vi "Periodic Tasks.vi"(8 "error in":errorcluster) -> ()   [LabVIEW 2016]
doc: "This VI runs in parallel to other tasks. It can contain as many user-defined periodic loops as you need. These can carry out PID or other sorts of timed response."
uses:
  <vilib>/Rock Robotics/WPI/Utilities/WPI_GetSetVariantRefNum.vi
  <vilib>/Instr/_visa.llb/VISA Configure Serial Port (Instr).vi
  2_11_17/Systems/Global 1.vi
panel:
  out "Drive L0 Effort":dbl format="%#_13g"
  out "Drive R0 Effort":dbl format="%#_13g"
  in  "off set":dbl=55.0 format="%#_13g"
  out "read buffer":string="B:3,X:197.00,Y:124.00"
  in  "Search_Params":string[](array[string])=["B", "X", "Y", "W1", "H1", "W2", "H2"]
  out "Last Complete Message":string="B:2,X:197.00,Y:124.00,W1:9,H1:24,W2:9,H2:23"
  out "length":i32=43
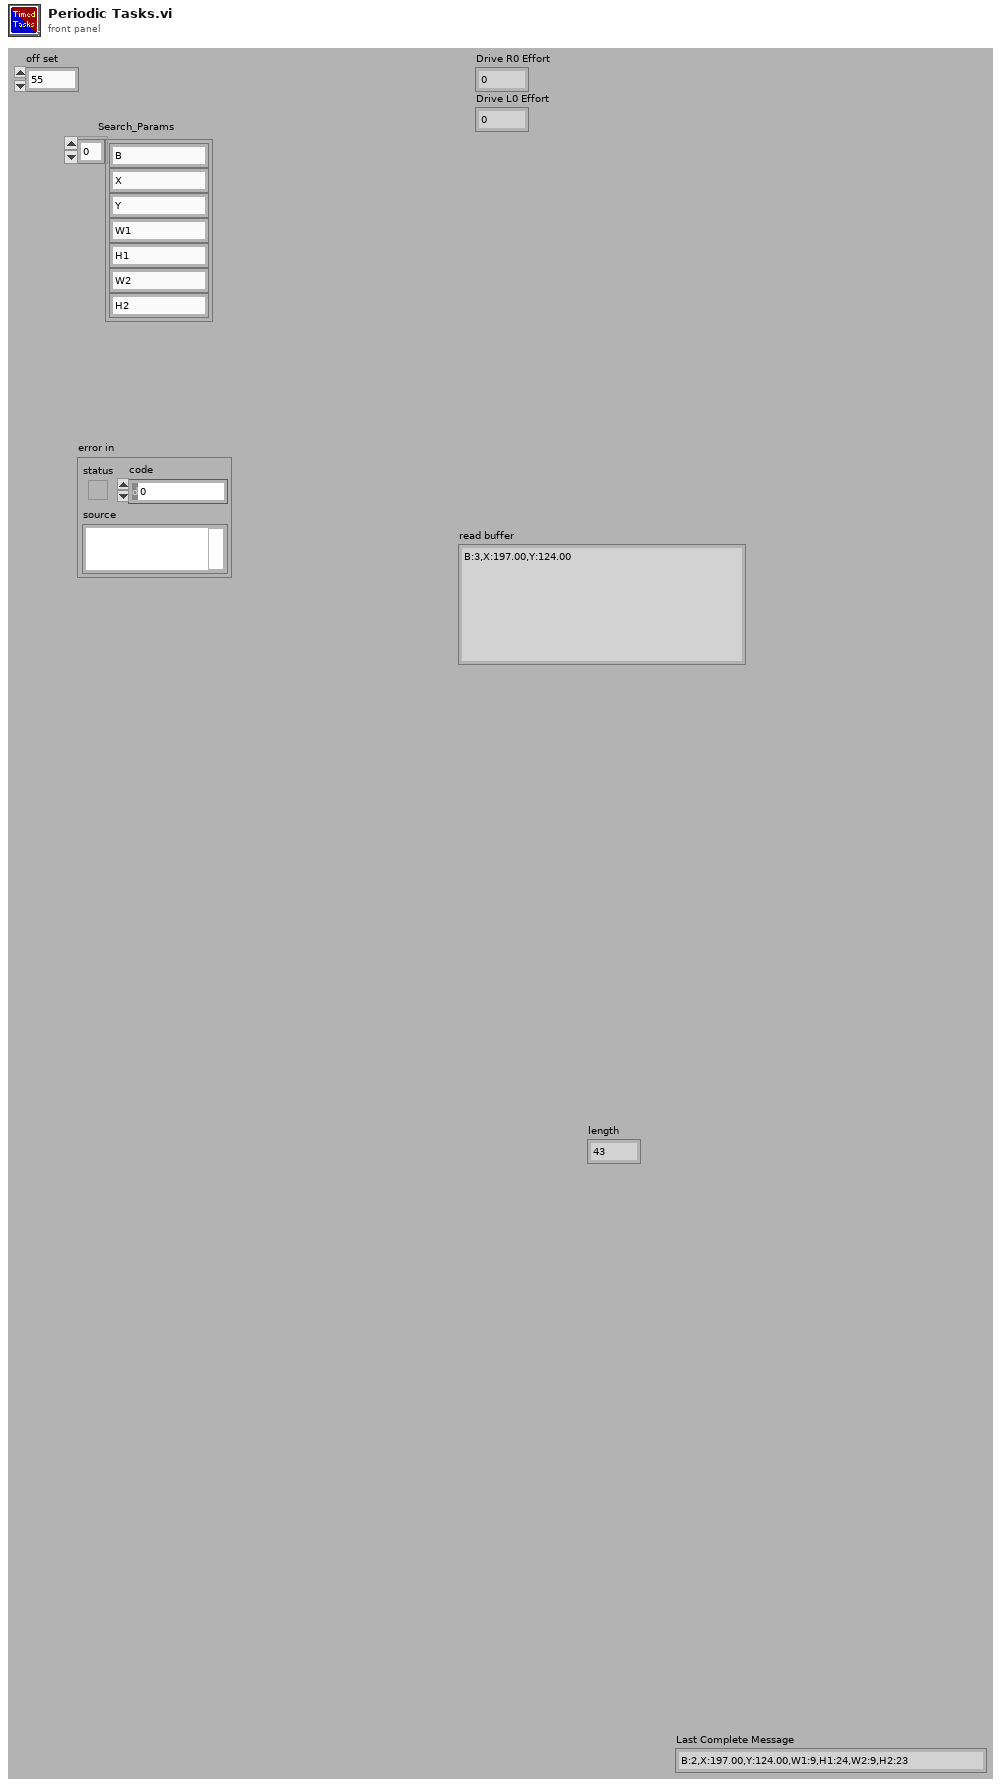
[diagram p1: front panel]
types:
  T1 = typedef "WPI_JoystickDevRef.ctl" = cluster{"Device":T2}
  T2 = typedef "WPI_JoystickDeviceEnum.ctl" = enum16{"USB 0", "USB 1", "USB 2", "USB 3", "USB 4", "USB 5"}
  T3 = typedef "WPI_MotorControlDeviceRef.ctl" = cluster{"DeviceStatus":errorcluster, "Type":T4, "PWM":cluster{"PWM Channel":T5, "DeadBand":T6}, "CAN":cluster{"Device Number":u8, "SetOutput VI Ref":variant, "GetOutput VI Ref":variant, "Enable VI Ref":variant, "Disable VI Ref":variant, "Data":variant}, "Invert":bool}
  T4 = typedef "WPI_MotorControlType.ctl" = enum16{"PWM", "CAN"}
  T5 = typedef "FPGA_DIOPWMChannel.ctl" = enum8{"PWM 0", "PWM 1", "PWM 2", "PWM 3", "PWM 4", "PWM 5", "PWM 6", "PWM 7", "PWM 8", "PWM 9", "PWM MXP 0", "PWM MXP 1", "PWM MXP 2", "PWM MXP 3", "PWM MXP 4", "PWM MXP 5", "PWM MXP 6", "PWM MXP 7", "PWM MXP 8", "PWM MXP 9", "Invalid"}
  T6 = typedef "WPI_PWMDeadband.ctl" = cluster{"Name":string, "maxPositivePwm":i32, "minPositivePwm":i32, "centerPwm":i32, "maxNegativePwm":i32, "minNegativePwm":i32, "angularRange":u16}
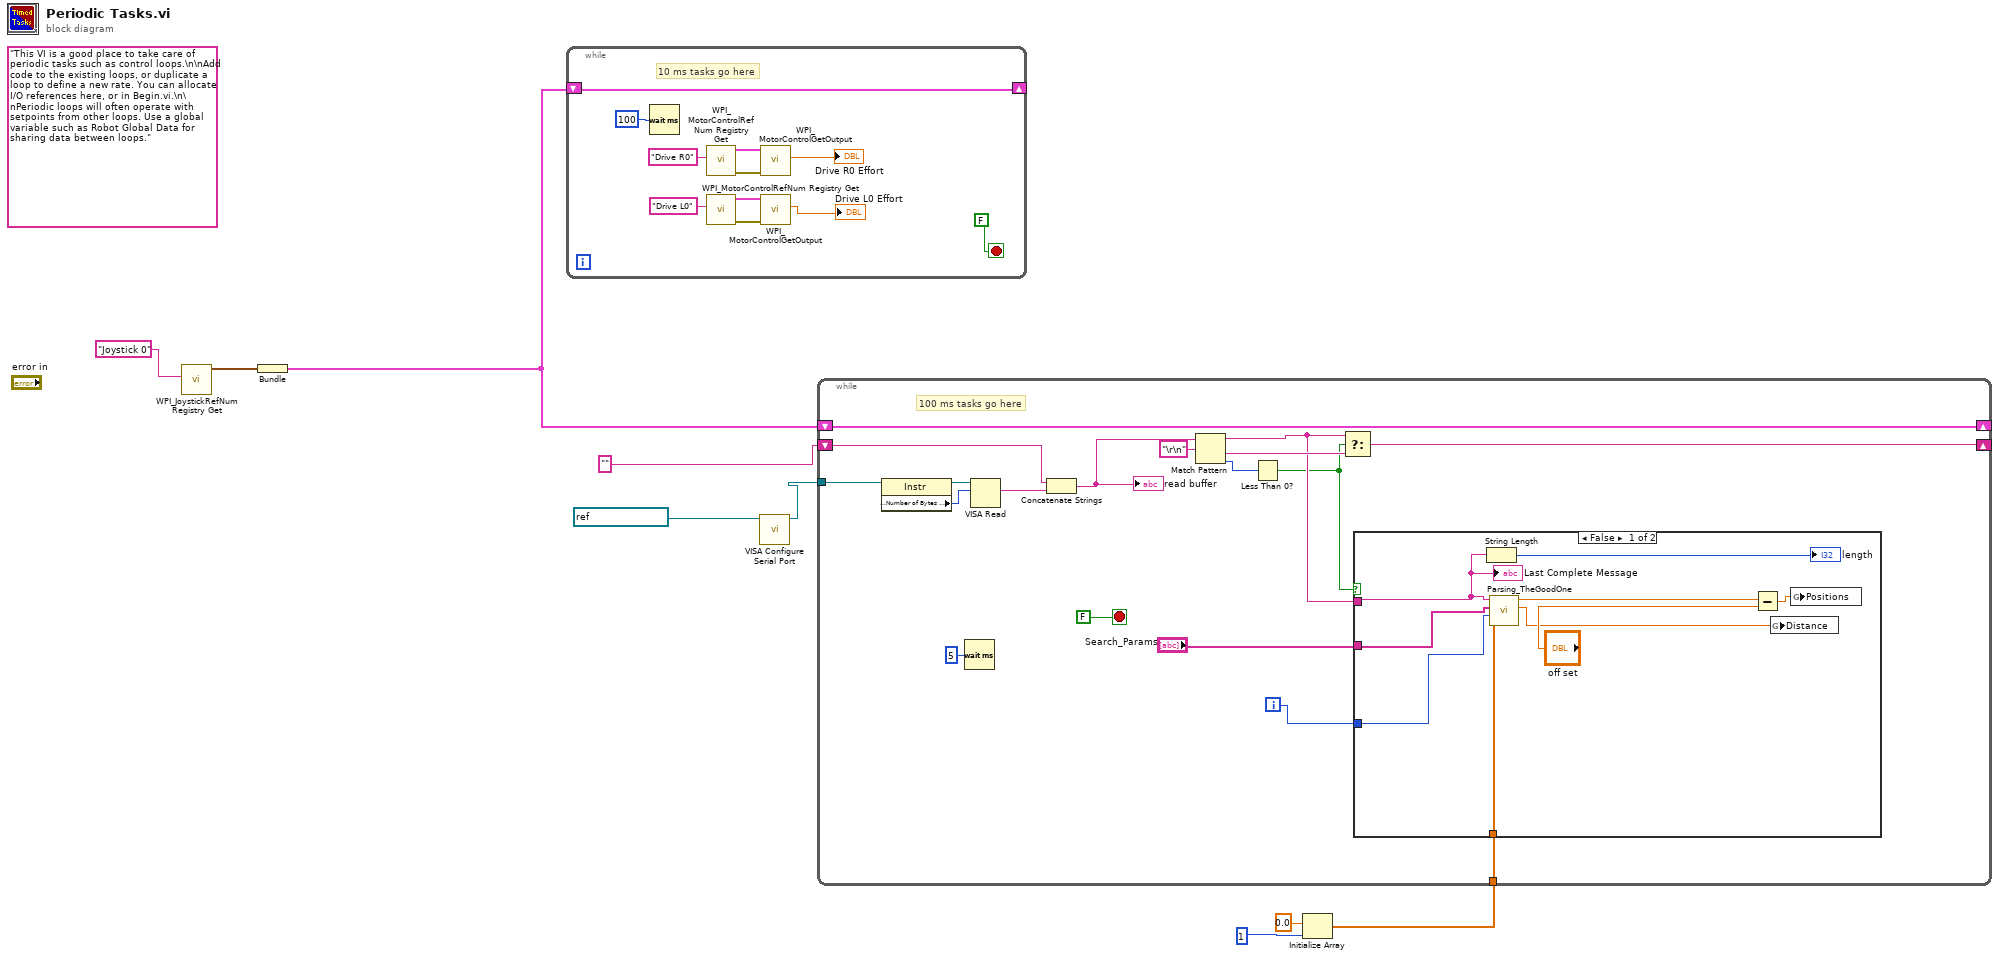
[diagram p0: block diagram]
diagram:
  (unwired) "This VI is a good place to take care of periodic tasks such as control loops.\n\nAdd code to the existing loops, or duplicate a loop to define a new rate. You can allocate I/O references here, or in Begin.vi.\n\nPeriodic loops will often operate with setpoints from other loops. Use a global variable such as Robot Global Data for sharing data between loops."
  n1 = call <vilib>:"WPI_JoystickRefNum Registry Get.vi"("refnum name"="Joystick 0") -> ("JoystickDevRef"=w8:T1)  [unwired: 1 in, 9 out]
  n2 = Bundle("JoystickDevRef"=w8) -> (w7:cluster{"JoystickDevRef":T1})  [unwired: 1 out]
  n3 = while {
    shift-right: [w18] -> _
    shift-left: w7 -> [w18]
    stop <- FALSE stop-if-true
    # "10 ms tasks go here"
    n4 = Wait (ms)(milliseconds to wait=u32 100) -> ()  [unwired: 1 out]
    n5 = call <vilib>:"WPI_MotorControlRefNum Registry Get.vi"("refnum name"="Drive R0") -> ("error out"=w13:errorcluster, "MotorControlDevRef"=w17:T3)  [unwired: 9 in]
    n6 = call <vilib>:"WPI_MotorControlRefNum Registry Get.vi"("refnum name"="Drive L0") -> ("error out"=w12:errorcluster, "MotorControlDevRef"=w14:T3)  [unwired: 9 in]
    n7 = call <vilib>:"WPI_MotorControlGetOutput.vi"("error in"=w13, "MotorControlDevRef"=w17) -> ("Output"=→"Drive R0 Effort":dbl)  [unwired: 7 in, 2 out]
    n8 = call <vilib>:"WPI_MotorControlGetOutput.vi"("error in"=w12, "MotorControlDevRef"=w14) -> ("Output"=→"Drive L0 Effort":dbl)  [unwired: 7 in, 2 out]
  }
  n9 = call-poly "VISA Configure Serial Port"("VISA resource name"=refnum<visa-resource-name> "ASRL2::INSTR") -> ("VISA resource name out"=w5:refnum<visa-resource-name>)  [unwired: 13 in, 1 out]
  n10 = Initialize Array(0.0 ("element"), 1) -> (w1:dbl[])
  n11 = while {
    shift-right: [w37] -> _
    shift-left: w7 -> [w37]
    tunnel: w5 -> [w32]
    shift-right: [w24] -> _
    shift-left: "" -> [w31]
    tunnel: w1 -> [w21]
    i -> [w22]
    stop <- FALSE stop-if-true
    # "100 ms tasks go here"
    n12 = property class="Instr"(reference=w32) -> (reference out=w36:refnum<visa-resource-name>, "Serial Settings:Number of Bytes at Serial Port"=w35:u32)  [unwired: 1 in, 1 out]
    n13 = Wait (ms)(milliseconds to wait=u32 5) -> ()  [unwired: 1 out]
    n14 = VISA Read(VISA resource name=w36, byte count=w35) -> (read buffer=w30:string)  [unwired: 1 in, 3 out]
    n15 = Concatenate Strings(w31, w30) -> (w29:string)
    "read buffer" <- w29
    n16 = Match Pattern(string=w29, regular expression="\r\n") -> (before substring=w25:string, after substring=w26:string, offset past match=w27:i32)  [unwired: 1 in, 1 out]
    n17 = Less Than 0?(x=w27) -> (x < 0?=w23:bool)
    n18 = Select(t=w25, s=w23, f=w26) -> (s? t:f=w24:string)
    n19 = case shown="False" w23 {
      tunnel: "Search_Params" -> [w46 _]
      tunnel: w25 -> [w45 _]
      tunnel: w22 -> [w40 _]
      tunnel: w21 -> [w39 _]
      frame False {
        n20 = String Length(string=w45) -> (length=→"length":i32)
        n21 = call "Parsing_TheGoodOne.vi"("array"=w39, "Iterations"=w40, "Search_Params"=w46, "Input"=w45) -> ("Corrected distance"=w41:dbl, "Value-Reference"=w44:dbl)  [unwired: 4 in]
        n22 = Subtract(x=w44, y="off set") -> (x-y=w42:dbl)
        n23 = global write "Global 1.vi" "Distance"(w41) -> ()
        n24 = global write "Global 1.vi" "Positions"(w42) -> ()
        "Last Complete Message" <- w45
      }
      frame True {
      }
    }
  }
